vi "PCSLauncher.panel.vi"(0 "object ref":refnum<vi>, 5 "error in (no error)":errorcluster) -> (19 "error out":errorcluster)   [LabVIEW 2014, in "PCSLauncher.lvlib"]
doc: "By this VI a ross relais can be monitored and switched. \n\nThe indicators \"CLOSED\", \"OPEN\" and \"SWITCH STATE\" show the value of the Beckhoff-Tag: blue indicates bad tag status reference problems, darkgreen false and lightgreen on. If everything is working fine, \"CLOSED\" and \"SWITCH STATE\" should show the same value, while \"OPEN\" has the opposite value. \n\nThe oval button switches the ross relais. It should be in the same state as the \"SWITCH STATE\" indicator. \n\n\"EXIT\" closes the front panel (GUI), while \"Delete Instance\" disconnects and removes the instance from the PCS.\n\nThis VI has no machine safety relevant logig: there is neither a check of internal conclict nor with other objects, for example conflict with other ross relais. Therefore it must be handled with care and should be operated by well educated operators only. It is forseen exclusively for direct operating and testing of the system. \n\nLicense Agreement for this software:\n\nCopyright (C)\nGesellschaft für Schwerionenforschung, GSI\nPlanckstr. 1\n64291 Darmstadt\nGermany\n\nContact: D.Beck@gsi.de \n\nThis program is free software; you can redistribute it and/or modify it under the terms of the GNU General Public License as published by the Free Software Foundation; either version 2 of the license, or (at your option) any later version.\n\nThis program is distributed in the hope that it will be useful, but WITHOUT ANYW ARRANTY; without even the implied warranty of MERCHANTABILITY or FITNESS FOR A PARTICULAR PURPOSE. See the GNU General License for more details (http://www.gnu.org).\n\nGesellschaft für Schwerionenforschung, GSI\nPlanckstr. 1, 64291 Darmstadt, Germany\nFor all questions and ideas contact: M.Richter@gsi.de, H.Brand@gsi.de or D.Beck@gsi.de.\nLast update: 18-DEC-2002"
uses:
  PCSLauncher.lvlib
  CSCore/CSObj/CSObj.lvlib
  PH_Common/PH_Common.lvlib
  PH_Class/PH_Class.lvlib
panel:
  out "uOPA":u32(colorbox) caption="Beckhoff"
  out "Max":u32(colorbox) caption="Beckhoff"
  out "PulsedPower-PA":u32(colorbox) caption="Beckhoff"
  in  "Launch PCS":bool
  out "Compressor":u32(colorbox) caption="Beckhoff"
  out "MAS":u32(colorbox) caption="Beckhoff"
  out "PA-Exit":u32(colorbox) caption="PP Beckhoff"
  out "Z6-Compressor":u32(colorbox) caption="Beckhoff"
  out "Z6-Southtower":u32(colorbox) caption="Beckhoff"
  in  "Delete":bool
  in  "Exit":bool
  out "ns-Frontend":u32(colorbox) caption="Beckhoff"
  out "fs-Frontend":u32(colorbox) caption="Beckhoff"
  out "Z6-Northtower":u32(colorbox) caption="PP Beckhoff"
  out "PA-Input":u32(colorbox) caption="Beckhoff"
  out "MainAmp":u32(colorbox) caption="Beckhoff"
  out "Shotdirector":u32(colorbox) caption="Beckhoff"
  out "Lila":u32(colorbox) caption="PP Beckhoff"
  out "PulsedPower":u32(colorbox) caption="Beckhoff"
  out "Experiment-Laserlabor":u32(colorbox) caption="Exp-LL"
  out "Experiment":u32(colorbox) caption="Beckhoff"
  out "Global":u32(colorbox) caption="Beckhoff"
  out "PILS":u32(colorbox) caption="Beckhoff"
  out "Timing":u32(colorbox) caption="Beckhoff"
  out "PulsedPower-Beckhoff":u32(colorbox) caption="PP Beckhoff"
  out "Beckhoff":u32(colorbox)
  # "PCS"
  # "3.40"
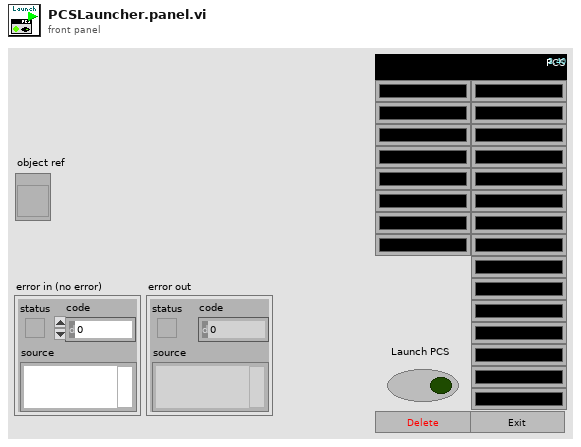
[diagram p1: front panel]
types:
  T1 = cluster{"GUI Ref":refnum<vi>, "Super alive?":bool, "Start-GOG alive?":bool}
  T2 = typedef "PCSLauncher.lvlib/PCSLauncher.i attribute.ctl" = cluster{"PCS Systems":cluster{"GUI Ref":refnum<vi>, "Super alive?":bool, "Start-GOG alive?":bool}[], "GUI Refs":cluster{"Delete":refnum<vi>, "Launch PCS":refnum<vi>}}
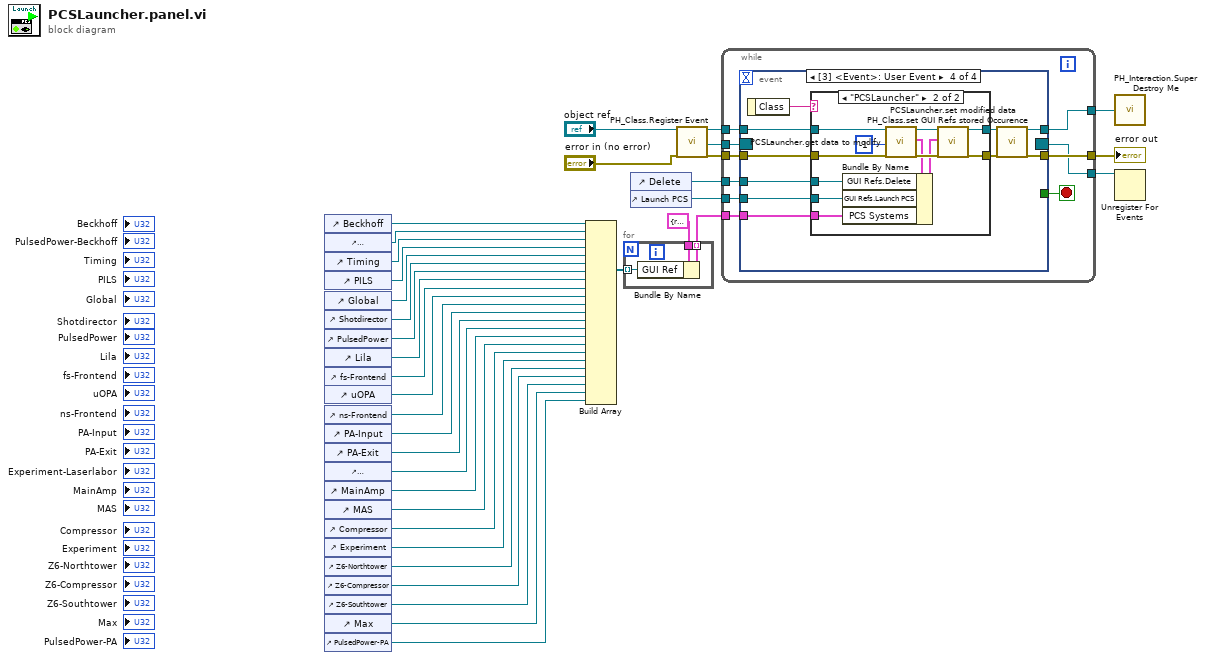
[diagram p0: block diagram]
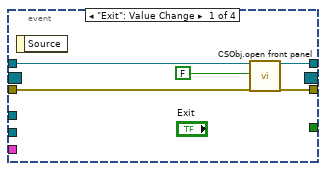
[diagram p2: hidden frame]
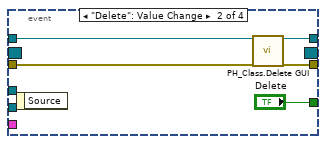
[diagram p3: hidden frame]
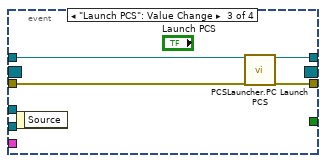
[diagram p4: hidden frame]
diagram:
  n1 = control-ref of="Beckhoff"() -> (w33:refnum<vi>)
  n2 = control-ref of="PulsedPower-Beckhoff"() -> (w31:refnum<vi>)
  n3 = control-ref of="Timing"() -> (w30:refnum<vi>)
  n4 = control-ref of="PILS"() -> (w29:refnum<vi>)
  n5 = control-ref of="Global"() -> (w28:refnum<vi>)
  n6 = control-ref of="Shotdirector"() -> (w27:refnum<vi>)
  n7 = control-ref of="PulsedPower"() -> (w26:refnum<vi>)
  n8 = control-ref of="Lila"() -> (w25:refnum<vi>)
  n9 = control-ref of="fs-Frontend"() -> (w24:refnum<vi>)
  n10 = control-ref of="uOPA"() -> (w10:refnum<vi>)
  n11 = control-ref of="ns-Frontend"() -> (w23:refnum<vi>)
  n12 = control-ref of="PA-Input"() -> (w22:refnum<vi>)
  n13 = control-ref of="PA-Exit"() -> (w21:refnum<vi>)
  n14 = control-ref of="Experiment-Laserlabor"() -> (w20:refnum<vi>)
  n15 = control-ref of="MainAmp"() -> (w19:refnum<vi>)
  n16 = control-ref of="MAS"() -> (w18:refnum<vi>)
  n17 = control-ref of="Compressor"() -> (w17:refnum<vi>)
  n18 = control-ref of="Experiment"() -> (w16:refnum<vi>)
  n19 = control-ref of="Z6-Northtower"() -> (w15:refnum<vi>)
  n20 = control-ref of="Z6-Compressor"() -> (w14:refnum<vi>)
  n21 = control-ref of="Z6-Southtower"() -> (w13:refnum<vi>)
  n22 = control-ref of="Max"() -> (w12:refnum<vi>)
  n23 = control-ref of="PulsedPower-PA"() -> (w11:refnum<vi>)
  n24 = Build Array(w33, w31, w30, w29, w28, w27, w26, w25, w24, w10, w23, w22, w21, w20, w19, w18, w17, w16, w15, w14, w13, w12, w11) -> (w32:refnum<vi>[])
  n25 = for {
    tunnel: T1 {"GUI Ref"=refnum, "Super alive?"=FALSE, "Start-GOG alive?"=FALSE} ("System") -> [w39]
    tunnel: w32 -> [w38] mode=indexing
    tunnel: [w37] -> w1 mode=indexing
    n26 = Bundle By Name(cluster=w39, "GUI Ref"=w38) -> (w37:T1)
  }
  n27 = control-ref of="Delete"() -> (w3:refnum<vi>)
  n28 = control-ref of="Launch PCS"() -> (w2:refnum<vi>)
  n29 = call "PH_Class.Register Event.vi"("i ref in"="object ref", "error in (no error)"="error in (no error)") -> ("i ref out"=w9:refnum<vi>, "Event Registration Refnum"=w7:refnum<event-registration>, "error out"=w8:errorcluster)  [unwired: 15 in]
  n30 = while {
    tunnel: w9 -> [w46]
    tunnel: [w45] -> w36
    tunnel: w8 -> [w48]
    tunnel: [w47] -> w35
    tunnel: w7 -> [w44]
    tunnel: [w43] -> w6
    tunnel: w3 -> [w42]
    tunnel: w2 -> [w41]
    tunnel: w1 -> [w40]
    stop <- w49 stop-if-true
    n31 = event shown="[3] <Event>: User Event" {
      selector: w44 -> [_ _ _ _]
      dyn-events: [_ _ _ _] -> w43
      timeout: _ -> [_ _ _ _]
      tunnel: [_ "Delete" _ _] -> w49
      tunnel: w46 -> [w54 w58 w63 w73]
      tunnel: w48 -> [w52 w57 w62 w70]
      tunnel: [w51 w56 w61 w68] -> w47
      tunnel: [w50 w55 w60 w71] -> w45
      tunnel: w42 -> [_ _ _ w66]
      tunnel: w41 -> [_ _ _ w65]
      tunnel: w40 -> [_ _ _ w64]
      event "Exit": Value Change {
        n32 = event-data() -> ()  [unwired: 1 in, 1 out]
        n33 = call "CSObj.open front panel.vi"("i ref in"=w54, "frontPanelOpen"=FALSE ("front panel open"), "error in (no error)"=w52) -> ("i ref out"=w50:refnum<vi>, "error out"=w51:errorcluster)  [unwired: 15 in]
      }
      event "Delete": Value Change {
        n34 = event-data() -> ()  [unwired: 1 in, 1 out]
        n35 = call "PH_Class.Delete GUI.vi"("VI in"=w58, "error in (no error)"=w57) -> ("VI out"=w55:refnum<vi>, "error out"=w56:errorcluster)  [unwired: 16 in]
      }
      event "Launch PCS": Value Change {
        n36 = event-data() -> ()  [unwired: 1 in, 1 out]
        n37 = call "PCSLauncher.PC Launch PCS.vi"("VI in"=w63, "error in (no error)"=w62) -> ("VI out"=w60:refnum<vi>, "error out"=w61:errorcluster)  [unwired: 16 in]
      }
      event User Event {
        n38 = event-data() -> ("Class"=w67:string)  [unwired: 1 in]
        n39 = case shown="\"PCSLauncher\"" w67 {
          tunnel: w73 -> [w75 w82]
          tunnel: [w75 w81] -> w72
          tunnel: w70 -> [w74 w80]
          tunnel: [w74 w79] -> w69
          tunnel: w66 -> [_ w78]
          tunnel: w65 -> [_ w77]
          tunnel: w64 -> [_ w76]
          frame Default {
          }
          frame "PCSLauncher" {
            n40 = call "PCSLauncher.get data to modify.vi"("i ref in"=w82, "ms timeout (10000)"=-1, "error in (no error)"=w80) -> ("i ref out"=w87:refnum<vi>, "i attribute"=w85:T2, "error out"=w86:errorcluster)  [unwired: 13 in, 1 out]
            n41 = Bundle By Name(cluster=w85, "GUI Refs.Delete"=w78, "GUI Refs.Launch PCS"=w77, "PCS Systems"=w76) -> (w84:T2)
            n42 = call "PCSLauncher.set modified data.vi"("i ref in"=w87, "i attribute"=w84, "error in (no error)"=w86) -> ("i ref out"=w81:refnum<vi>, "error out"=w79:errorcluster)  [unwired: 15 in]
          }
        }
        n43 = call "PH_Class.set GUI Refs stored Occurence.vi"("i ref in"=w72, "error in (no error)"=w69) -> ("i ref out"=w71:refnum<vi>, "error out"=w68:errorcluster)  [unwired: 16 in]
      }
    }
  }
  "error out" <- w35
  n44 = call "PH_Interaction.Super Destroy Me.vi"("i ref out"=w36) -> ()
  n45 = Unregister For Events(event registration refnum=w6) -> ()  [unwired: 1 in, 1 out]
